vi "quasiquote_eval.vi"(10 "Environment in":T1, 11 "Expression in":T2) -> (2 "Environment out":T1, 3 "Expression out":T2)   [LabVIEW 2020]
uses:
  ExpressionType.ctl
  Expression.ctl
  Environment.ctl
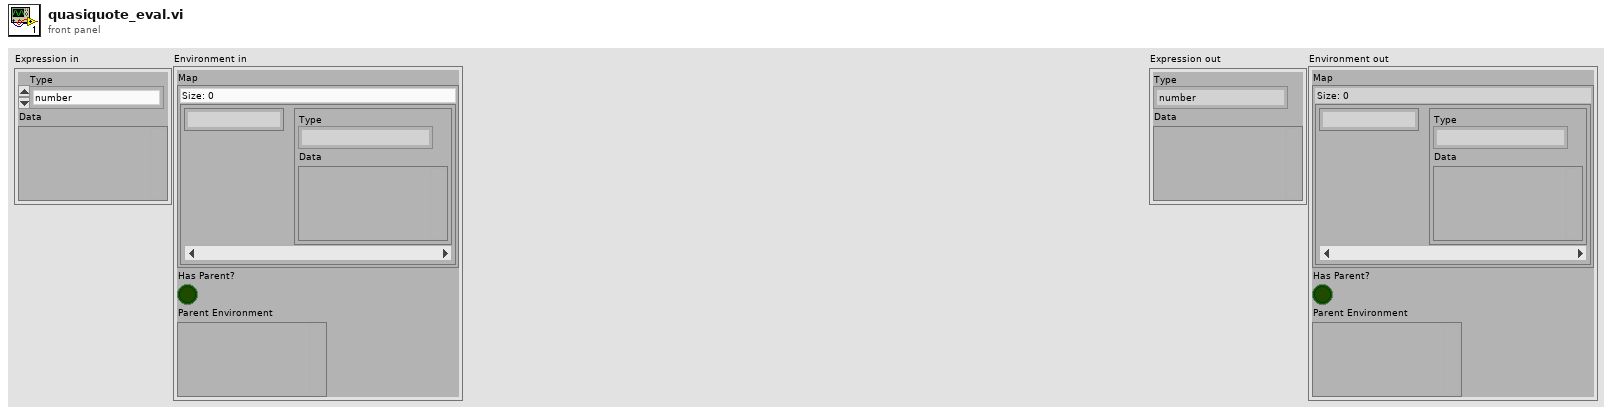
[diagram p1: front panel]
types:
  T1 = typedef "Environment.ctl" = cluster{"Map":map{string, T2}, "Has Parent?":bool, "Parent Environment":variant}
  T2 = typedef "Expression.ctl" = cluster{"Type":T3, "Data":variant}
  T3 = typedef "ExpressionType.ctl" = enum16{"number", "string", "symbol", "primitive", "list", "closure", "macro", "nil", "error"}
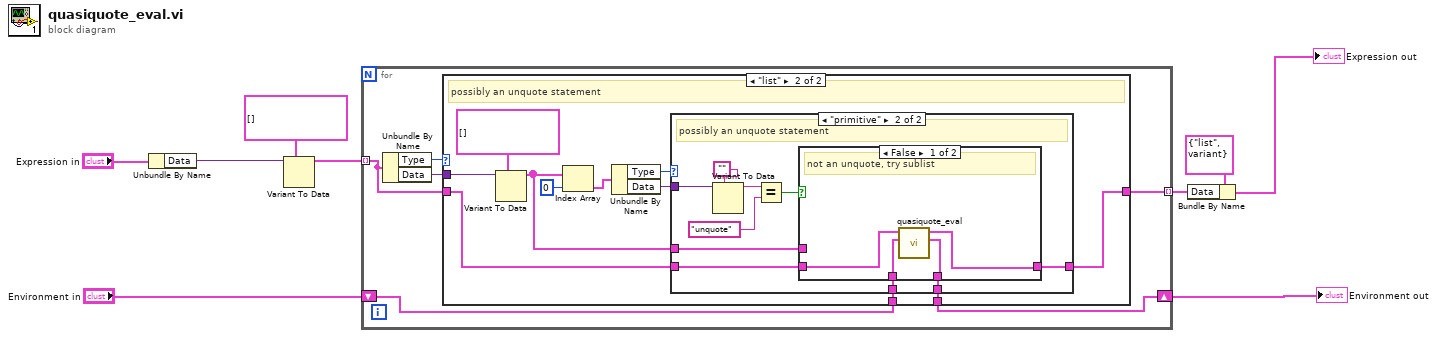
[diagram p0: block diagram]
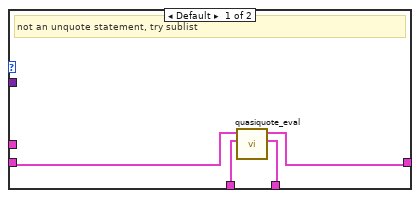
[diagram p3: hidden frame]
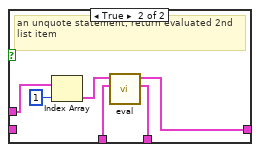
[diagram p4: hidden frame]
diagram:
  n1 = Unbundle By Name("Expression in") -> ("Data"=w9:variant)
  n2 = Variant To Data(type=T2[] [], Variant=w9) -> (data=w3:T2[])  [unwired: 1 in, 1 out]
  n3 = for {
    tunnel: w3 -> [w13] mode=indexing
    shift-right: [w10] -> w6
    shift-left: "Environment in" -> [w11]
    tunnel: [w14] -> w1 mode=indexing
    n4 = Unbundle By Name(w13) -> ("Type"=w15:T3, "Data"=w12:variant)
    n5 = case shown="\"list\"" w15 {
      tunnel: [w17 w22] -> w14
      tunnel: w13 -> [w17 w23]
      tunnel: w12 -> [_ w27]
      tunnel: w11 -> [w16 w19]
      tunnel: [w16 w18] -> w10
      frame Default {
        # "for sure not an unquote statement, pass data without evaluating"
      }
      frame "list" {
        # "possibly an unquote statement"
        n6 = Variant To Data(type=T2[] [], Variant=w27) -> (data=w21:T2[])  [unwired: 1 in, 1 out]
        n7 = Index Array(array=w21, index=0) -> (element=w25:T2)
        n8 = Unbundle By Name(w25) -> ("Type"=w24:T3, "Data"=w20:variant)
        n9 = case shown="\"primitive\"" w24 {
          tunnel: w23 -> [w29 w37]
          tunnel: [w30 w36] -> w22
          tunnel: w21 -> [_ w35]
          tunnel: w20 -> [_ w39]
          tunnel: w19 -> [w32 w34]
          tunnel: [w31 w33] -> w18
          frame Default {
            # "not an unquote statement, try sublist"
            n10 = call "quasiquote_eval.vi"("Environment in"=w32, "Expression in"=w29) -> ("Environment out"=w31:T1, "Expression out"=w30:T2)  [unwired: 8 in]
          }
          frame "primitive" {
            # "possibly an unquote statement"
            n11 = Variant To Data(type="", Variant=w39) -> (data=w42:string)  [unwired: 1 in, 1 out]
            n12 = Equal?(x=w42, y="unquote") -> (x = y?=w38:bool)
            n13 = case shown="False" w38 {
              tunnel: w37 -> [w44 _]
              tunnel: [w43 w47] -> w36
              tunnel: w35 -> [_ w50]
              tunnel: w34 -> [w46 w49]
              tunnel: [w45 w48] -> w33
              frame False {
                # "not an unquote, try sublist"
                n14 = call "quasiquote_eval.vi"("Environment in"=w46, "Expression in"=w44) -> ("Environment out"=w45:T1, "Expression out"=w43:T2)  [unwired: 8 in]
              }
              frame True {
                # "an unquote statement, return evaluated 2nd list item"
                n15 = Index Array(array=w50, index=1) -> (element=w51:T2)
                n16 = call "eval.vi"("Environment in"=w49, "Expression in"=w51) -> ("Environment out"=w48:T1, "Expression out"=w47:T2)  [unwired: 6 in]
              }
            }
          }
        }
      }
    }
  }
  "Environment out" <- w6
  n17 = Bundle By Name(cluster=T2 {"Type"=enum."list", "Data"=variant} ("Expression in"), "Data"=w1) -> (→"Expression out":T2)
